vi "Hatch State Control.vi"(2 "Elevator State":string, 3 "Vacuum Pump Power":dbl) -> ()   [LabVIEW 2018]
uses:
  RefNumsDriverStation.vi
  Robot States.vi
panel:
  in  "Vacuum Pump Off Time (ms)":u32=2000
  in  "Hatch Eject Time (ms)":u32=1000
  in  "Suction Cup Pulse (ms)":u32=100
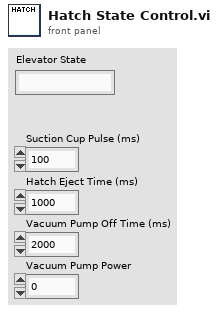
[diagram p1: front panel]
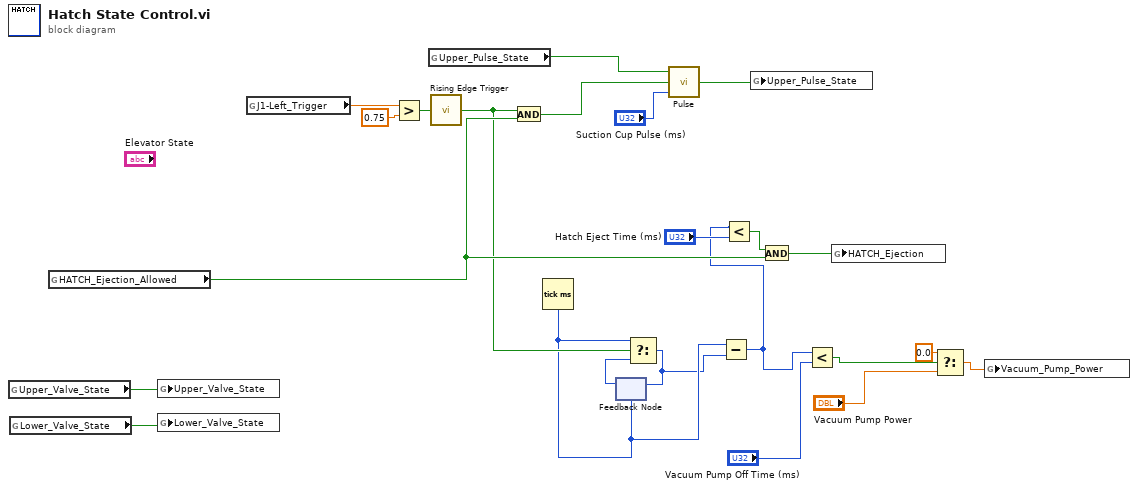
[diagram p0: block diagram]
diagram:
  n1 = global read "Robot States.vi" "Upper_Valve_State"() -> (w2:bool)
  n2 = global read "Robot States.vi" "Lower_Valve_State"() -> (w1:bool)
  n3 = global read "Robot States.vi" "HATCH_Ejection_Allowed"() -> (w16:bool)
  n4 = global write "Robot States.vi" "Upper_Valve_State"(w2) -> ()
  n5 = global write "Robot States.vi" "Lower_Valve_State"(w1) -> ()
  n6 = global read "RefNumsDriverStation.vi" "J1-Left_Trigger"() -> (w23:dbl)
  n7 = Greater?(x=w23, y=0.75) -> (0:w21:bool)
  n8 = global read "Robot States.vi" "Upper_Pulse_State"() -> (w20:bool)
  n9 = call "Rising Edge Trigger.vi"("Raw Signal"=w21) -> ("Trigger"=w15:bool)
  n10 = And(x=w15, y=w16) -> (x .and. y?=w19:bool)
  n11 = Tick Count (ms)() -> (millisecond timer value=w13:u32)
  n12 = feedback #1(w13) -> (w14:u32)
  n13 = Select(t=w13, s=w15, f=w14) -> (s? t:f=w12:u32)
  n14 = feedback-in #1(w12) -> ()
  n15 = call "Pulse.vi"("Pulse_Durration (ms)"="Suction Cup Pulse (ms)", "Trigger"=w19, "State_In"=w20) -> ("State_Out"=w17:bool)  [unwired: 2 in]
  n16 = Subtract(x=w13, y=w12) -> (x-y=w3:u32)
  n17 = Less?(x=w3, y="Hatch Eject Time (ms)") -> (x < y?=w5:bool)
  n18 = global write "Robot States.vi" "Upper_Pulse_State"(w17) -> ()
  n19 = And(x=w5, y=w16) -> (x .and. y?=w6:bool)
  n20 = Less?(x=w3, y="Vacuum Pump Off Time (ms)") -> (x < y?=w10:bool)
  n21 = global write "Robot States.vi" "HATCH_Ejection"(w6) -> ()
  n22 = Select(t=0.0, s=w10, f="Vacuum Pump Power") -> (s? t:f=w9:dbl)
  n23 = global write "Robot States.vi" "Vacuum_Pump_Power"(w9) -> ()
